vi "testGetTelElement.vi"(8 "error in (no error)":errorcluster) -> (0 "error out":errorcluster)   [LabVIEW 2018]
doc: "Test the getTelElement.vi"
uses:
  src/TcpServer/TcpServer.lvclass
  src/TcpServer/TcpServer.lvclass/TcpServer.ctl
  src/TcpServerTel/TcpServerTel.lvclass/TcpServerTel.ctl
  <vilib>/addons/_JKI Toolkits/Caraya/classes/Assert/Assert Equal Value_Variant.vi
  src/TcpServerTel/TcpServerTel.lvclass
  <vilib>/addons/_JKI Toolkits/Caraya/classes/Test/Test.lvclass
  <vilib>/addons/_JKI Toolkits/Caraya/classes/Assert/Assert.lvclass
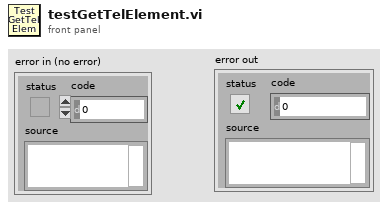
[diagram p1: front panel]
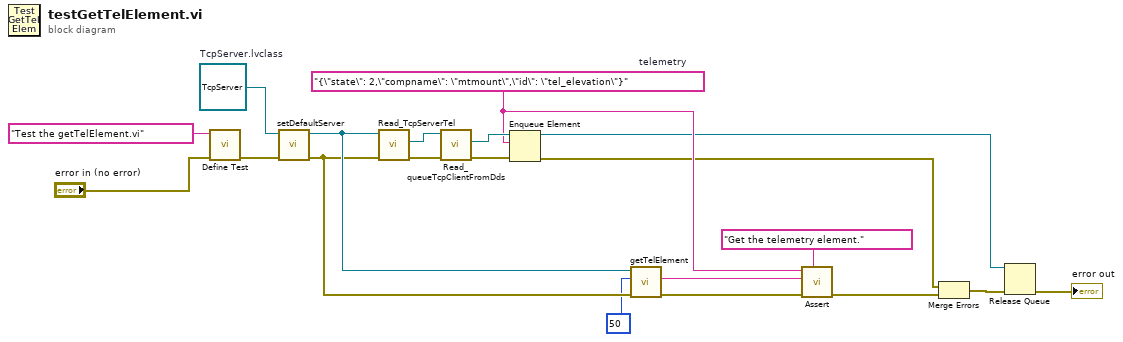
[diagram p0: block diagram]
diagram:
  w7 = "{\"state\": 2,\"compname\": \"mtmount\",\"id\": \"tel_elevation\"}"  # telemetry
  w17 = refnum<class "TcpServer.lvclass"> refnum  # TcpServer.lvclass
  n1 = call <vilib>:"Define Test.vi"("error in (no error)"="error in (no error)", "Label (VI Title)"="Test the getTelElement.vi") -> ("error out"=w19:errorcluster)  [unwired: 9 in]
  n2 = call "setDefaultServer.vi"("error in (no error)"=w19, "TcpServer.lvclass"=w17) -> ("error out"=w9:errorcluster, "tcpServer out"=w10:refnum<class "TcpServer.lvclass">)  [unwired: 8 in]
  n3 = call "Read_TcpServerTel.vi"("error in (no error)"=w9, "TcpServer in"=w10) -> ("error out"=w13:errorcluster, "TcpServerTel.lvclass"=w14:refnum<class "TcpServerTel.lvclass">)  [unwired: 7 in, 1 out]
  n4 = call "Read_queueTcpClientFromDds.vi"("error in (no error)"=w13, "TcpServerTel in"=w14) -> ("error out"=w12:errorcluster, "queueTcpClientFromDds"=w11:refnum<queue>)  [unwired: 7 in, 1 out]
  n5 = Enqueue Element(queue=w11, element=w7, error in (no error)=w12) -> (queue out=w3:refnum<queue>, error out=w1:errorcluster)  [unwired: 1 in, 1 out]
  n6 = call "getTelElement.vi"("error in (no error)"=w9, "telQueueServerTimeout"=50, "TcpServer in"=w10) -> ("error out"=w5:errorcluster, "tcpPacket"=w6:string)  [unwired: 5 in, 2 out]
  n7 = call-poly <vilib>:"Assert.vi"("Label"="Get the telemetry element.", "error in (no error)"=w5, "Y"=w6, "X"=w7) -> ("error out"=w15:errorcluster)  [unwired: 7 in]
  n8 = Merge Errors(w1, w15) -> (w2:errorcluster)
  n9 = Release Queue(queue=w3, error in (no error)=w2) -> (error out=→"error out":errorcluster)  [unwired: 1 in, 2 out]
